vi "Create.vi"(8 "error in (no error)":errorcluster) -> (0 "error out":errorcluster, 3 "Ignore Inputs Comparator":refnum<class "Ignore Inputs Comparator.lvclass">)   [LabVIEW 2020, in "Ignore Inputs Comparator.lvclass"]
uses:
  Ignore Inputs Comparator.lvclass
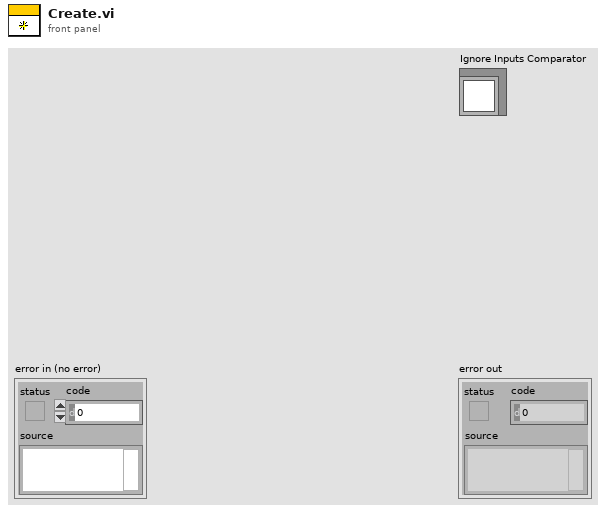
[diagram p1: front panel]
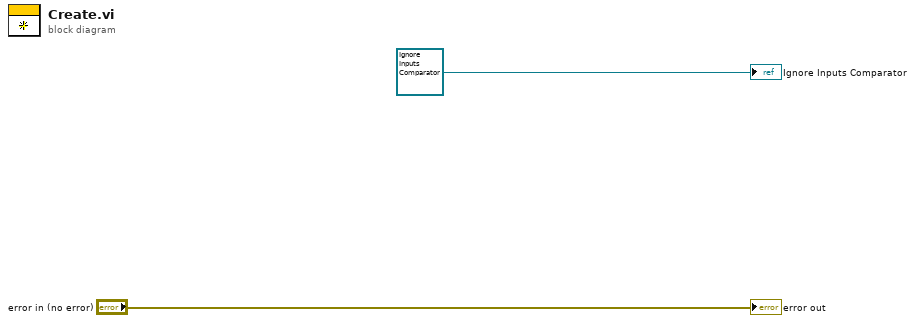
[diagram p0: block diagram]
diagram:
  "error out" <- "error in (no error)"
  "Ignore Inputs Comparator" <- refnum<class "Ignore Inputs Comparator.lvclass"> refnum ("Ignore Inputs Comparator")
